vi "CSTK_Enum_Creator_SaveTemporaryControlVI.vi"(8 "错误输入（无错误）":errorcluster, 11 "VI输入":refnum<vi>) -> (0 "错误输出":errorcluster, 2 "存储路径输出":path)   [LabVIEW 2015, in "CSTK_Enum Creator.lvlib"]
uses:
  CSTK_Enum Creator.lvlib
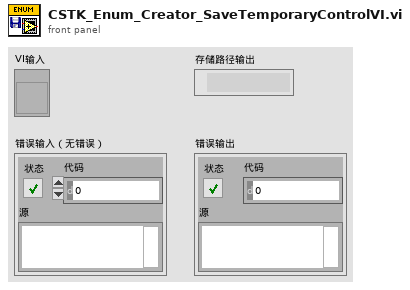
[diagram p1: front panel]
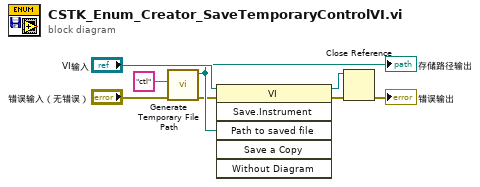
[diagram p0: block diagram]
diagram:
  n1 = call <vilib>:"Generate Temporary File Path.vi"("error in (no error)"="错误输入（无错误）", "Temporary File Extension (tmp)"="ctl") -> ("error out"=w1:errorcluster, "Unique Temporary File Path"=w7:path)  [unwired: 8 in]
  "存储路径输出" <- w7
  n2 = invoke class="VI" method="Save.Instrument"(reference="VI输入", error in=w1, "Path to saved file"=w7) -> (reference out=w5:refnum<vi>, error out=w4:errorcluster)  [unwired: 3 in, 4 out]
  n3 = Close Reference(reference=w5, error in (no error)=w4) -> (error out=→"错误输出":errorcluster)
